vi "DFS Data - Replace Node.vi"(8 "Error In":errorcluster, 9 "Node Index":i32, 10 "New Node Value":T2, 11 "DFS Data In":T1) -> (0 "Error Out":errorcluster, 3 "DFS Data Out":T1)   [LabVIEW 2022 SP3]
doc: "<add documentation here>"
uses:
  DFS Data (cluster).ctl
  DFS Node (cluster).ctl
  DFS Child Node (cluster).ctl
panel:
  # "Development\nControls or indicators that are useful for development or testing, but which are not outputs of the VI."
  # "Input\nInputs to the VI"
  # "Output\nOutputs of the VI"
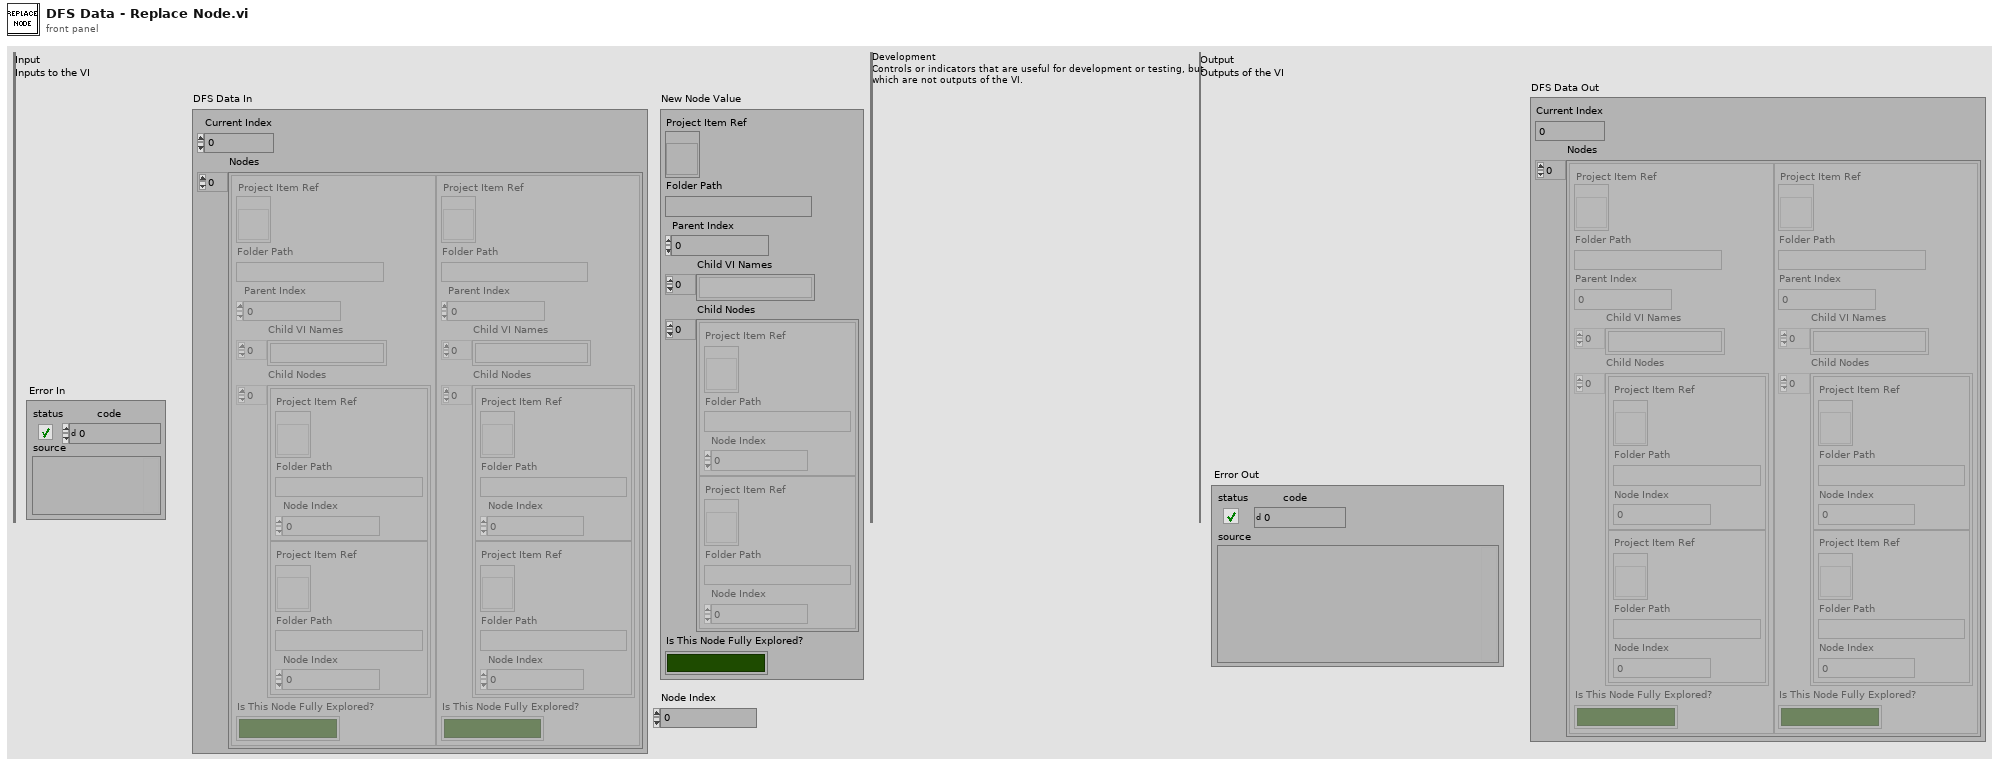
[diagram p1: front panel]
types:
  T1 = typedef "DFS Data (cluster).ctl" = cluster{"Current Index":i32, "Nodes":T2[]}
  T2 = typedef "DFS Node (cluster).ctl" = cluster{"Project Item Ref":refnum<vi>, "Folder Path":string, "Parent Index":i32, "Child VI Names":string[], "Child Nodes":T3[], "Is This Node Fully Explored?":bool}
  T3 = typedef "DFS Child Node (cluster).ctl" = cluster{"Project Item Ref":refnum<vi>, "Folder Path":string, "Node Index":i32}
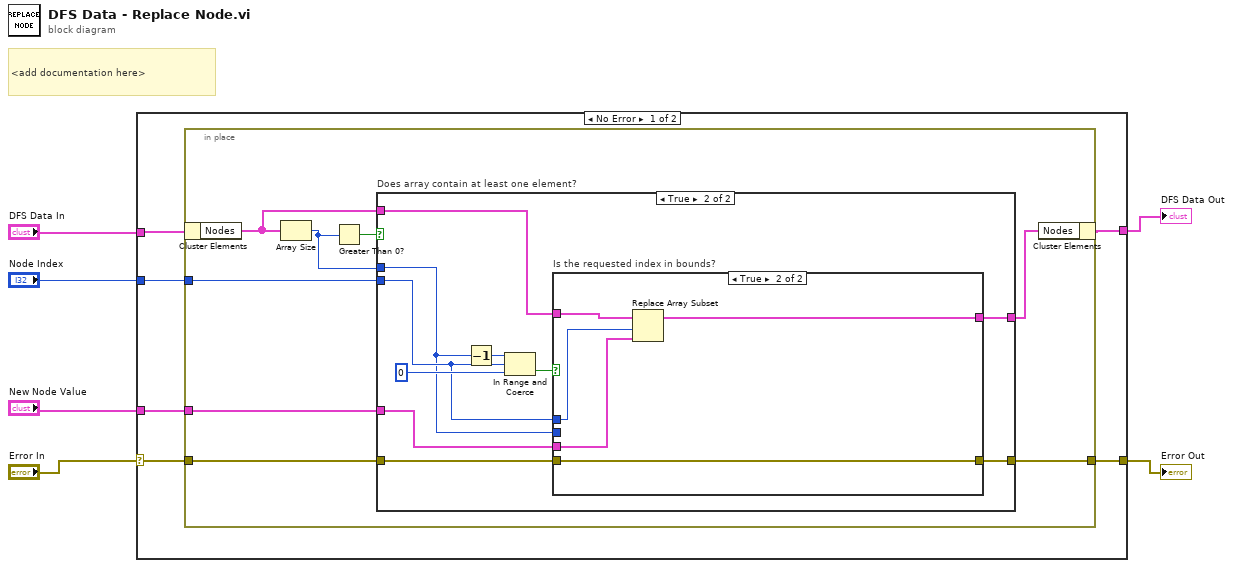
[diagram p0: block diagram]
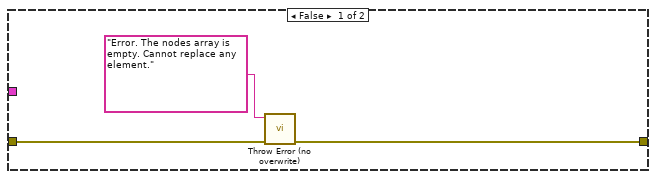
[diagram p2: hidden frame]
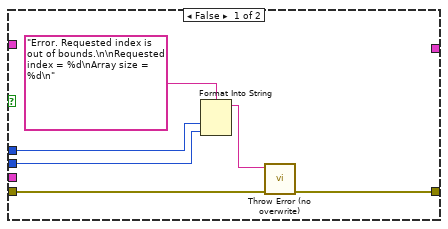
[diagram p3: hidden frame]
diagram:
  # "<add documentation here>"
  n1 = case shown="No Error" "Error In" {
    selector: "Error In" -> [w12 w46]
    tunnel: [w11 w46] -> w5
    tunnel: "Node Index" -> [w10 _]
    tunnel: "DFS Data In" -> [w8 w45]
    tunnel: "New Node Value" -> [w9 _]
    tunnel: [w7 w45] -> w1
    frame No Error {
      n2 = in-place {
        in-place-border: w12 -> [w20]
        in-place-border: [w19] -> w11
        in-place-border: w10 -> [w17]
        in-place-border: w9 -> [w15]
        n3 = in-place-cluster #1(w8) -> ("Nodes"=w14:T2[])
        n4 = Array Size(array=w14) -> (size(s)=w16:i32)
        n5 = Greater Than 0?(x=w16) -> (x > 0?=w18:bool)
        n6 = case "Does array contain at least one element?" shown="True" w18 {
          tunnel: w20 -> [w23 w31]
          tunnel: [w22 w30] -> w19
          tunnel: w17 -> [_ w28]
          tunnel: w16 -> [_ w27]
          tunnel: w14 -> [_ w26]
          tunnel: [_ w25] -> w13
          tunnel: w15 -> [_ w24]
          frame False {
            n7 = call "Throw Error (no overwrite).vi"("error in"=w23, "Error Message"="Error. The nodes array is empty. Cannot replace any element.") -> ("error out"=w22:errorcluster)  [unwired: 9 in]
          }
          frame True {
            n8 = Decrement(x=w27) -> (x-1=w32:i32)
            n9 = In Range and Coerce(upper limit=w32, x=w28, lower limit=0) -> (In Range?=w29:bool)  [unwired: 1 out]
            n10 = case "Is the requested index in bounds?" shown="True" w29 {
              tunnel: w31 -> [w39 w44]
              tunnel: [w38 w44] -> w30
              tunnel: w28 -> [w35 w42]
              tunnel: w27 -> [w34 _]
              tunnel: w26 -> [_ w43]
              tunnel: [_ w41] -> w25
              tunnel: w24 -> [_ w40]
              frame False {
                n11 = Format Into String(format string="Error. Requested index is out of bounds.\n\nRequested index = %d\nArray size = %d\n", w35, w34) -> (resulting string=w36:string)  [unwired: 2 in, 1 out]
                n12 = call "Throw Error (no overwrite).vi"("error in"=w39, "Error Message"=w36) -> ("error out"=w38:errorcluster)  [unwired: 9 in]
              }
              frame True {
                n13 = Replace Array Subset "Replace Array Subset"(array=w43, new element=w40, index=w42) -> (w41:T2[])
              }
            }
          }
        }
        n14 = in-place-cluster #1("Nodes"=w13) -> (w7:T1)
      }
    }
    frame Error {
    }
  }
  "Error Out" <- w5
  "DFS Data Out" <- w1
